vi "RT Stop.vi"() -> ()   [LabVIEW 2014]
panel:
  in  "RT Stop":bool
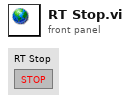
[diagram p1: front panel]
diagram:
